vi "RESTART.vi"() -> ()   [LabVIEW 2015]
uses:
  <vilib>/Utility/miscctls.llb/LVPointTypeDef.ctl
  <vilib>/Utility/config.llb/NI_LVConfig.lvlib
  <vilib>/zip/NI_Unzip.lvlib
panel:
  out "Note":string
  in  "File Infor":cluster{"File name":string, "Time":timestamp}
  in  "Note Error":string
  out "filenames":string[](array[string])
  out "FileInfor":cluster{"File name":string, "Time":timestamp}[](array[cluster])
  out "max time":timestamp
  out "error out":errorcluster
  in  "Duong dan server":string="\\\\192.168.1.5\\data\\EN\\1. UPDATE\\KIEM KE"
  # "RESTARTING..."
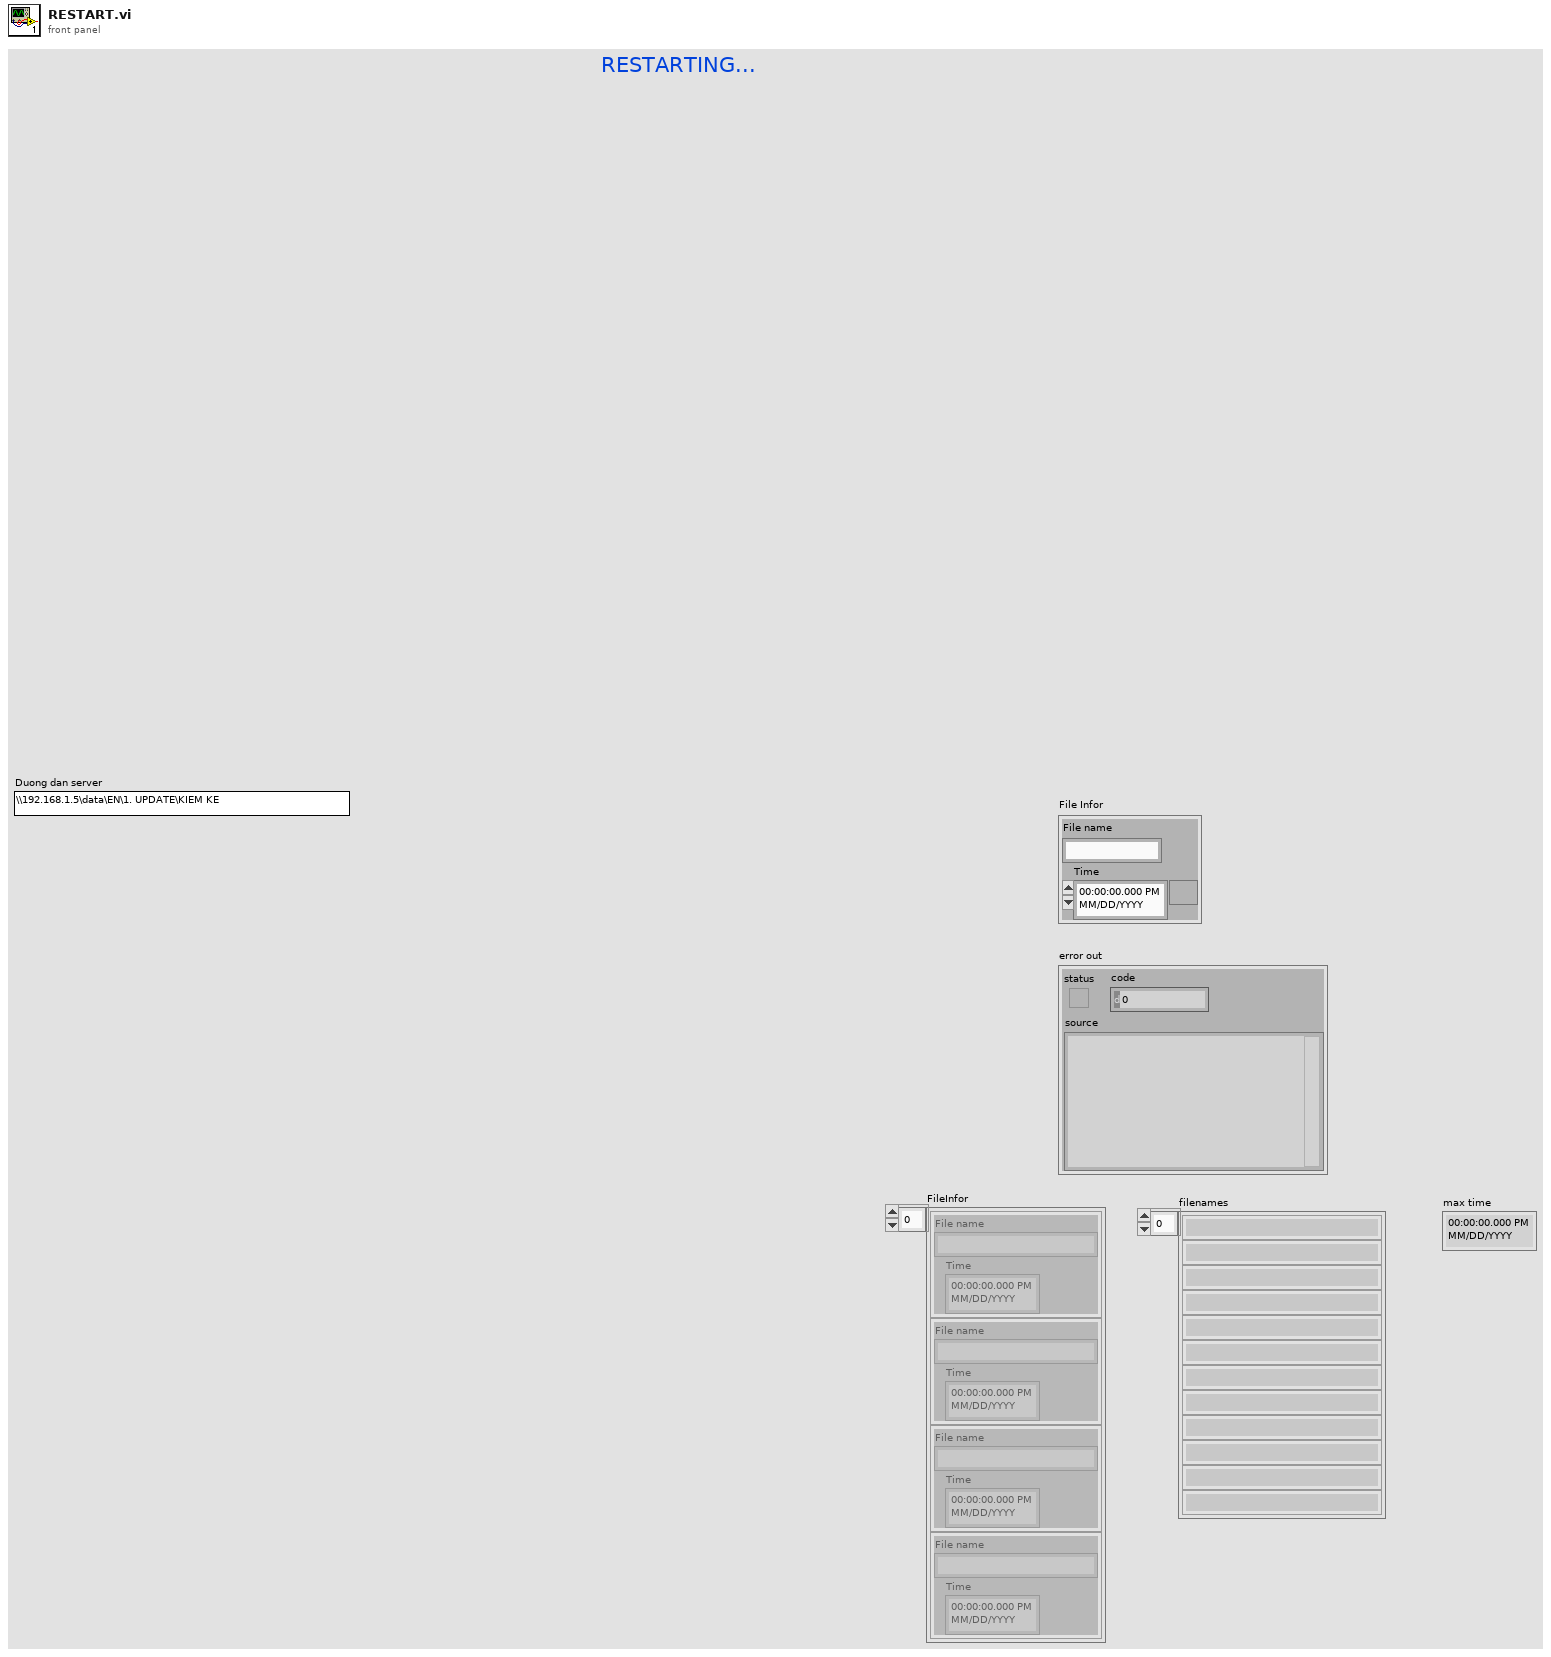
[diagram p1: front panel]
types:
  T1 = typedef "LVPointTypeDef.ctl" = cluster{"Horizontal":i16, "Vertical":i16}
  T2 = typedef "NI_LVConfig.lvlib/Config Data RefNum.ctl" = refnum<k1>
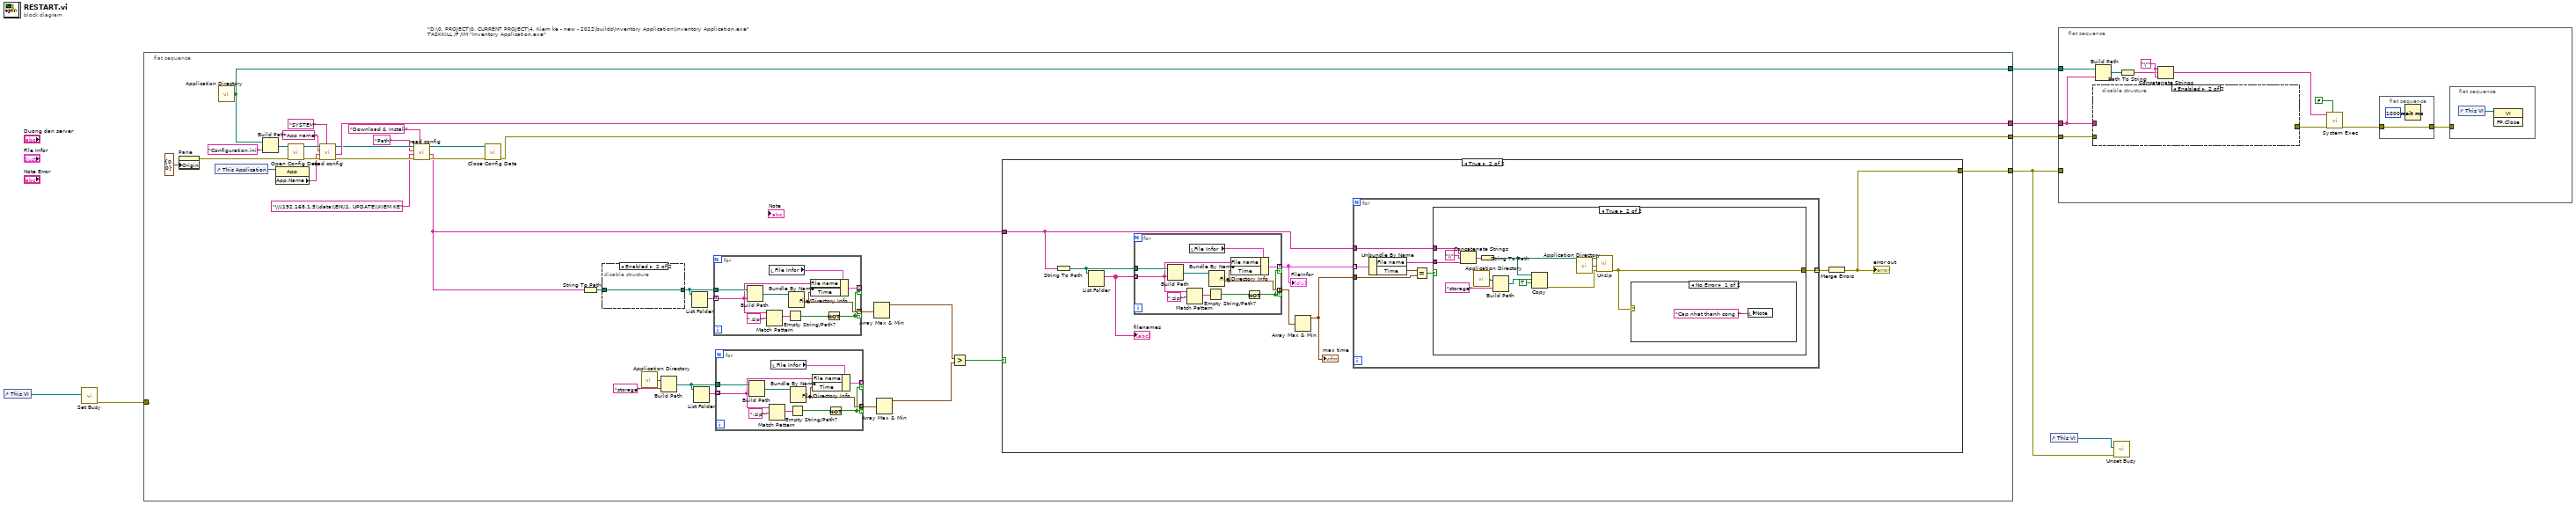
[diagram p0: block diagram]
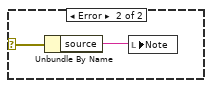
[diagram p4: hidden frame]
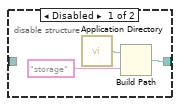
[diagram p5: hidden frame]
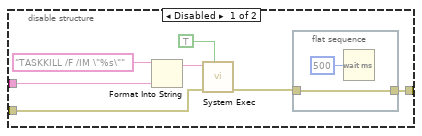
[diagram p6: hidden frame]
diagram:
  # "\"D:\\0. PROJECT\\0. CURRENT PROJECT\\4. Kiem ke - new - 2022\\builds\\Inventory Application\\Inventory Application.exe\"\nTASKKILL /F /IM \"Inventory Application.exe\""
  n1 = control-ref of="This VI"() -> (w4:refnum<vi>)
  n2 = call <vilib>:"Set Busy.vi"("VI reference (current VI)"=w4) -> ("error out"=w3:errorcluster)  [unwired: 9 in, 1 out]
  n3 = flat-sequence {
    tunnel: [w33] -> w7
    tunnel: [w32] -> w6
    tunnel: [w31] -> w5
    tunnel: [w9] -> w2
    tunnel: [w8] -> _
    tunnel: w3 -> [w8]
    frame #0 {
      n4 = property on="Pane" class="Pane"("Origin"=T1 {"Horizontal"=0, "Vertical"=0}) -> (error out=w30:errorcluster)  [unwired: 2 in, 1 out]
      n5 = control-ref of="This Application"() -> (w35:refnum<vi>)
      n6 = call <vilib>:"Application Directory.vi"() -> ("Application Directory"=w33:path)
      n7 = Build Path(base path=w33, name or relative path="Configuration.ini") -> (appended path=w40:path)
      n8 = property class="App"(reference=w35) -> ("App.Name"=w34:string)  [unwired: 1 in, 2 out]
      n9 = call <vilib>:"Open Config Data.vi"("error in (no error)"=w30, "configuration file path"=w40) -> ("error out"=w38:errorcluster, "refnum"=w41:T2)  [unwired: 7 in, 1 out]
      n10 = call "read config.vi"("Section"="SYSTEM", "error in (no error) 2"=w38, "Default value"=w34, "Key"="App name", "refnum"=w41) -> ("error out"=w28:errorcluster, "value"=w32:string, "refnum out"=w29:T2)  [unwired: 4 in]
      n11 = call "read config.vi"("Section"="Download & Install", "error in (no error) 2"=w28, "Default value"="\\\\192.168.1.5\\data\\EN\\1. UPDATE\\KIEM KE", "Key"="Path", "refnum"=w29) -> ("error out"=w26:errorcluster, "value"=w10:string, "refnum out"=w27:T2)  [unwired: 4 in]
      n12 = call <vilib>:"Close Config Data.vi"("error in (no error)"=w26, "refnum"=w27) -> ("error out"=w31:errorcluster)  [unwired: 8 in, 1 out]
      n13 = String To Path(string=w10) -> (path=w14:path)
      n14 = disable-structure shown="Enabled" {
        disable-tunnel: [w93 w96] -> w13
        disable-tunnel: w14 -> [_ w96]
        frame Disabled {
          n15 = call <vilib>:"Application Directory.vi"() -> ("Application Directory"=w95:path)
          n16 = Build Path(base path=w95, name or relative path="storage") -> (appended path=w93:path)
        }
        frame Enabled {
        }
      }
      n17 = call <vilib>:"Application Directory.vi"() -> ("Application Directory"=w17:path)
      n18 = Build Path(base path=w17, name or relative path="storage") -> (appended path=w15:path)
      n19 = List Folder(path=w13) -> (filenames=w12:string[])  [unwired: 3 in, 3 out]
      n20 = List Folder(path=w15) -> (filenames=w16:string[])  [unwired: 3 in, 3 out]
      n21 = for {
        tunnel: w12 -> [w100] mode=indexing
        tunnel: w13 -> [w106]
        tunnel: [w103] -> _ mode=indexing if=w97
        tunnel: [w102] -> w20 mode=indexing if=w97
        n22 = Build Path(base path=w106, name or relative path=w100) -> (appended path=w105:path)
        n23 = Match Pattern(string=w100, regular expression=".zip") -> (match substring=w98:string)  [unwired: 1 in, 3 out]
        n24 = local read "File Infor"() -> (w104:cluster{"File name":string, "Time":timestamp})
        n25 = Empty String/Path?(string/path=w98) -> (empty?=w99:bool)
        n26 = File/Directory Info(path=w105) -> (last mod=w102:timestamp)  [unwired: 1 in, 6 out]
        n27 = Bundle By Name(cluster=w104, "File name"=w100, "Time"=w102) -> (w103:cluster{"File name":string, "Time":timestamp})
        n28 = Not(x=w99) -> (.not. x?=w97:bool)
      }
      n29 = for {
        tunnel: w16 -> [w86] mode=indexing
        tunnel: w15 -> [w92]
        tunnel: [w89] -> _ mode=indexing if=w83
        tunnel: [w88] -> w19 mode=indexing if=w83
        n30 = Build Path(base path=w92, name or relative path=w86) -> (appended path=w91:path)
        n31 = Match Pattern(string=w86, regular expression=".zip") -> (match substring=w84:string)  [unwired: 1 in, 3 out]
        n32 = local read "File Infor"() -> (w90:cluster{"File name":string, "Time":timestamp})
        n33 = Empty String/Path?(string/path=w84) -> (empty?=w85:bool)
        n34 = File/Directory Info(path=w91) -> (last mod=w88:timestamp)  [unwired: 1 in, 6 out]
        n35 = Bundle By Name(cluster=w90, "File name"=w86, "Time"=w88) -> (w89:cluster{"File name":string, "Time":timestamp})
        n36 = Not(x=w85) -> (.not. x?=w83:bool)
      }
      n37 = Array Max & Min(array=w20) -> (max value=w22:timestamp)  [unwired: 3 out]
      n38 = Array Max & Min(array=w19) -> (max value=w21:timestamp)  [unwired: 3 out]
      n39 = Greater?(x=w22, y=w21) -> (0:w11:bool)
      n40 = case shown="True" w11 {
        tunnel: w10 -> [_ w44]
        tunnel: [_ w43] -> w9
        frame False {
        }
        frame True {
          n41 = String To Path(string=w44) -> (path=w46:path)
          n42 = List Folder(path=w46) -> (filenames=w45:string[])  [unwired: 3 in, 3 out]
          "filenames" <- w45
          n43 = for {
            tunnel: w45 -> [w76] mode=indexing
            tunnel: w46 -> [w82]
            tunnel: [w79] -> w47 mode=indexing if=w73
            tunnel: [w78] -> w48 mode=indexing if=w73
            n44 = Build Path(base path=w82, name or relative path=w76) -> (appended path=w81:path)
            n45 = Match Pattern(string=w76, regular expression=".zip") -> (match substring=w74:string)  [unwired: 1 in, 3 out]
            n46 = local read "File Infor"() -> (w80:cluster{"File name":string, "Time":timestamp})
            n47 = Empty String/Path?(string/path=w74) -> (empty?=w75:bool)
            n48 = File/Directory Info(path=w81) -> (last mod=w78:timestamp)  [unwired: 1 in, 6 out]
            n49 = Bundle By Name(cluster=w80, "File name"=w76, "Time"=w78) -> (w79:cluster{"File name":string, "Time":timestamp})
            n50 = Not(x=w75) -> (.not. x?=w73:bool)
          }
          "FileInfor" <- w47
          n51 = Array Max & Min(array=w48) -> (max value=w49:timestamp)  [unwired: 3 out]
          "max time" <- w49
          n52 = for {
            tunnel: w47 -> [w54] mode=indexing
            tunnel: w44 -> [w56]
            tunnel: [w55] -> w50 mode=indexing
            tunnel: w49 -> [w52]
            n53 = Unbundle By Name(w54) -> ("File name"=w57:string, "Time"=w53:timestamp)
            n54 = Equal?(x=w53, y=w52) -> (x = y?=w51:bool)
            n55 = case shown="True" w51 {
              tunnel: w57 -> [_ w69]
              tunnel: w56 -> [_ w67]
              tunnel: [_ w64] -> w55
              frame False {
              }
              frame True {
                n56 = Concatenate Strings(w67, "\\" ("string"), w69) -> (w66:string)
                n57 = call <vilib>:"Application Directory.vi"() -> ("Application Directory"=w62:path)
                n58 = String To Path(string=w66) -> (path=w63:path)
                n59 = Build Path(base path=w62, name or relative path="storage") -> (appended path=w60:path)
                n60 = Copy(9:TRUE ("overwrite (F)"), 10:w60, 11:w63) -> (0:w58:errorcluster)  [unwired: 2 in, 2 out]
                n61 = call <vilib>:"Application Directory.vi"() -> ("Application Directory"=w65:path)
                n62 = call <vilib>:"Unzip.vi"("error in (no error)"=w58, "Target directory (same as Zip file if empty)"=w65, "Zip file"=w63) -> ("error out"=w64:errorcluster)  [unwired: 6 in, 2 out]
                n63 = case shown="No Error" w64 {
                  selector: w64 -> [_ w72]
                  frame No Error {
                    n64 = local write "Note"("Cap nhat thanh cong !" ("Note Error")) -> ()
                  }
                  frame Error {
                    n65 = Unbundle By Name(w72) -> ("source"=w71:string)
                    n66 = local write "Note"(w71) -> ()
                  }
                }
              }
            }
          }
          n67 = Merge Errors(w50) -> (w43:errorcluster)
          "error out" <- w43
        }
      }
    }
  }
  n68 = control-ref of="This VI"() -> (w1:refnum<vi>)
  n69 = flat-sequence {
    tunnel: w7 -> [w109]
    tunnel: w6 -> [w108]
    tunnel: w5 -> [w107]
    tunnel: w2 -> [_]
    frame #0 {
      w115 = "\""
      n70 = disable-structure shown="Enabled" {
        disable-tunnel: w108 -> [w121 _]
        disable-tunnel: [w119 _] -> w111
        disable-tunnel: w107 -> [w118 _]
        frame Disabled {
          n71 = Format Into String(format string="TASKKILL /F /IM \"%s\"" ("command line"), w121) -> (resulting string=w122:string)  [unwired: 2 in, 1 out]
          n72 = call <vilib>:"System Exec.vi"("wait until completion? (T)"=TRUE, "error in (no error)"=w118, "command line"=w122) -> ("error out"=w120:errorcluster)  [unwired: 5 in, 3 out]
          n73 = flat-sequence {
            tunnel: [w125] -> w119
            tunnel: w120 -> [w125]
            frame #0 {
              n74 = Wait (ms)(milliseconds to wait=u32 500) -> ()  [unwired: 1 out]
            }
          }
        }
        frame Enabled {
        }
      }
      n75 = Build Path(base path=w109, name or relative path=w108) -> (appended path=w116:path)
      n76 = Path To String(path=w116) -> (string=w114:string)
      n77 = Concatenate Strings(w115, w114, w115) -> (w112:string)
      n78 = call <vilib>:"System Exec.vi"("wait until completion? (T)"=FALSE, "error in (no error)"=w111, "command line"=w112) -> ("error out"=w110:errorcluster)  [unwired: 5 in, 3 out]
      n79 = flat-sequence {
        tunnel: w110 -> [w127]
        tunnel: [w127] -> w117
        frame #0 {
          n80 = Wait (ms)(milliseconds to wait=u32 1000) -> ()  [unwired: 1 out]
        }
      }
      n81 = flat-sequence {
        tunnel: w117 -> [_]
        frame #0 {
          n82 = control-ref of="This VI"() -> (w129:refnum<vi>)
          n83 = invoke class="VI" method="FP.Close"(reference=w129) -> ()  [unwired: 2 in, 3 out]
        }
      }
    }
  }
  n84 = call <vilib>:"Unset Busy.vi"("error in (no error)"=w2, "VI reference (current VI)"=w1) -> ()  [unwired: 9 in, 1 out]
